vi "Main.vi"() -> ()   [LabVIEW 2018] (continued)
            n2414 = Not(x=w322) -> (.not. x?=→"ST90通讯状态":bool)
            n2415 = Index Array(array=w319, index=0 ("索引")) -> (element=w320:u32)
            n2416 = Number To Boolean Array(number=w320) -> (Boolean array=w321:bool[])
            n2417 = Index Array(array=w321, index #1=0 ("索引")) -> (element #1=w285:bool, element #2=w284:bool, element #3=w283:bool, element #4=w282:bool, element #5=w278:bool)  [unwired: 4 in]
            "ST901扫码请求" <- w285
            "ST901数据读取" <- w284
            "ST902扫码请求" <- w282
            "ST902数据读取" <- w278
            "ST901编码请求" <- w283
            n2418 = call <vilib>:"Boolean Crossing PtByPt.vi"("direction"=enum16{"either", "false-true", "true-false"}."false-true", "input"=w285) -> ("crossing"=w307:bool)  [unwired: 1 in]
            n2419 = disable-structure shown="启用" {
              disable-tunnel: [w334 w336] -> w294
              disable-tunnel: w285 -> [w333 w336]
              frame Disabled {
                n2420 = call <vilib>:"Boolean Crossing PtByPt.vi"("direction"=enum16{"either", "false-true", "true-false"}."true-false", "input"=w333) -> ("crossing"=w334:bool)  [unwired: 1 in]
              }
              frame Enabled {
              }
            }
            n2421 = case shown="真" w307 {
              tunnel: w309 -> [w513 w518]
              tunnel: w308 -> [w512 w519]
              tunnel: [w513 w517] -> w306
              tunnel: [w512 w515] -> w305
              frame False {
              }
              frame True {
                w527 = u16 0 items=["byte", "word", "Dword"] ("数据类型")
                w525 = u8 132 items=["I/O (P)"=128, "Input (I)"=129, "Output (Q)"=130, "Bit Memory (M)"=131, "Data (DB)"=132, "Instance Data (DI)"=133, "Local Data (L)"=134, "Predecessor Local Data (VL)"=135] ("寄存器类型")
                n2422 = call "S7_Read.vi"("TCP"=w518, "DB #"=u16 20, "读取长度"=u16 13, "寄存器类型"=w525, "起始地址"=u32 6, "数据类型"=w527, "error in"=w519) -> ("TCP"=w517:refnum<k5>, "数据"=w522:u32[], "error out"=w520:errorcluster)  [unwired: 5 in, 1 out]
                n2423 = To Unsigned Word Integer(number=w522) -> (unsigned 16bit integer=w521:u16[])
                n2424 = call "还原为字符串.vi"("error in (no error)"=w520, "输入数组"=w521) -> ("error out"=w516:errorcluster, "字符串"=w514:string)  [unwired: 8 in]
                n2425 = stacked-sequence {
                  tunnel: w516 -> [_ w531]
                  tunnel: [_ w530] -> w515
                  tunnel: w514 -> [w528 _]
                  frame #0 {
                    "901二维码" <- w528
                  }
                  frame #1 {
                    n2426 = property on="ST901扫码请求（事件）" class="Bool (严格)"(error in=w531, "Val(Sgnl)"=TRUE ("值(信号)")) -> (error out=w530:errorcluster)  [unwired: 1 in, 1 out]
                  }
                }
              }
            }
            n2427 = case shown="假" w294 {
              frame False {
                n2428 = local write "901扫码回复输入"(FALSE ("301扫码回复输入")) -> ()
              }
              frame True {
              }
            }
            n2429 = call <vilib>:"Boolean Crossing PtByPt.vi"("direction"=enum16{"either", "false-true", "true-false"}."false-true", "input"=w284) -> ("crossing"=w303:bool)  [unwired: 1 in]
            n2430 = disable-structure shown="启用" {
              disable-tunnel: enum16{"either", "false-true", "true-false"}."true-false" ("direction") -> [w343 _]
              disable-tunnel: [w342 w344] -> w300
              disable-tunnel: w284 -> [w341 w344]
              frame Disabled {
                n2431 = call <vilib>:"Boolean Crossing PtByPt.vi"("direction"=w343, "input"=w341) -> ("crossing"=w342:bool)  [unwired: 1 in]
              }
              frame Enabled {
              }
            }
            n2432 = case shown="真" w303 {
              tunnel: [w443 w460] -> w298
              tunnel: [w442 w445] -> w297
              tunnel: w305 -> [w442 w470]
              tunnel: w306 -> [w443 w471]
              frame False {
              }
              frame True {
                w467 = u16 2 items=["byte", "word", "Dword"] ("数据类型")
                w465 = u8 132 items=["I/O (P)"=128, "Input (I)"=129, "Output (Q)"=130, "Bit Memory (M)"=131, "Data (DB)"=132, "Instance Data (DI)"=133, "Local Data (L)"=134, "Predecessor Local Data (VL)"=135] ("寄存器类型")
                w480 = u16 2 items=["byte", "word", "Dword"] ("数据类型")
                w482 = u8 132 items=["I/O (P)"=128, "Input (I)"=129, "Output (Q)"=130, "Bit Memory (M)"=131, "Data (DB)"=132, "Instance Data (DI)"=133, "Local Data (L)"=134, "Predecessor Local Data (VL)"=135] ("寄存器类型")
                w475 = u16 1 items=["byte", "word", "Dword"] ("数据类型")
                w477 = u8 132 items=["I/O (P)"=128, "Input (I)"=129, "Output (Q)"=130, "Bit Memory (M)"=131, "Data (DB)"=132, "Instance Data (DI)"=133, "Local Data (L)"=134, "Predecessor Local Data (VL)"=135] ("寄存器类型")
                n2433 = call "S7_Read.vi"("TCP"=w471, "DB #"=u16 20, "读取长度"=u16 1, "寄存器类型"=w477, "起始地址"=u32 82, "数据类型"=w475, "error in"=w470) -> ("TCP"=w488:refnum<k5>, "数据"=w490:u32[], "error out"=w489:errorcluster)  [unwired: 5 in, 1 out]
                n2434 = Index Array(array=w490) -> (element=w492:u32)  [unwired: 1 in]
                n2435 = Equal?(x=w492, y=u32 1) -> (x = y?=w491:bool)
                n2436 = case shown="真" w491 {
                  tunnel: ["NG" "OK"] -> w469
                  frame False {
                  }
                  frame True {
                  }
                }
                n2437 = call "S7_Read.vi"("TCP"=w488, "DB #"=u16 20, "读取长度"=u16 12, "寄存器类型"=w482, "起始地址"=u32 34, "数据类型"=w480, "error in"=w489) -> ("TCP"=w462:refnum<k5>, "数据"=w458:u32[], "error out"=w461:errorcluster)  [unwired: 5 in, 1 out]
                n2438 = Divide(x=w458, y=u32[] [100, 100, 100, 100, 100, 100, 100, 100, 100, 100, 100, 100]) -> (x/y=w457:dbl[])
                n2439 = Number To Fractional String(number=w457, precision (6)=i16 2 ("精度(6)")) -> (F-format string=w468:string[])  [unwired: 2 in]
                n2440 = call "S7_Read.vi"("TCP"=w462, "DB #"=u16 20, "读取长度"=u16 9, "寄存器类型"=w465, "起始地址"=u32 100, "数据类型"=w467, "error in"=w461) -> ("TCP"=w460:refnum<k5>, "数据"=w454:u32[], "error out"=w459:errorcluster)  [unwired: 5 in, 1 out]
                n2441 = Divide(x=w454, y=u32[] [100, 100, 1000, 1000, 1000, 1000, 1000, 1000, 1000]) -> (x/y=w452:dbl[])
                n2442 = Delete From Array(array=w452, length=2 ("长度"), index=0 ("索引")) -> (deleted portion=w448:dbl[], array with subset deleted=w449:dbl[])
                n2443 = for {
                  tunnel: w449 -> [w509] mode=indexing
                  tunnel: [w508] -> w446 mode=indexing
                  n2444 = Number To Fractional String(number=w509, precision (6)=i16 3 ("精度(6)")) -> (F-format string=w508:string)  [unwired: 2 in]
                }
                n2445 = for {
                  tunnel: w448 -> [w506] mode=indexing
                  tunnel: [w504] -> w447 mode=indexing
                  n2446 = Number To Fractional String(number=w506, precision (6)=i16 2 ("精度(6)")) -> (F-format string=w504:string)  [unwired: 2 in]
                }
                n2447 = Format Date/Time String(time format string (%c)="%Y-%m-%d" ("时间格式字符串(%c)")) -> (date/time string=w493:string)  [unwired: 2 in]
                n2448 = Get Date/Time String(want seconds? (F)=TRUE ("需要秒？(F)")) -> (time string=w494:string)  [unwired: 2 in, 1 out]
                n2449 = Insert Into Array(array=string[] [] ("数组"), index=0 ("索引"), new element #1="901" ("新元素/子数组"), new element #2=w469, new element #3=w493, new element #4=w494, new element #5=w469, new element #6=w468, new element #7=w447, new element #8=w446) -> (w444:string[])
                n2450 = stacked-sequence {
                  tunnel: w459 -> [_ w499]
                  tunnel: [_ w496] -> w445
                  tunnel: w444 -> [w495 _]
                  frame #0 {
                    "901数据" <- w495
                  }
                  frame #1 {
                    n2451 = property on="ST901数据读取（事件）" class="Bool (严格)"(error in=w499, "Val(Sgnl)"=TRUE ("值(信号)")) -> (error out=w497:errorcluster)  [unwired: 1 in, 1 out]
                    n2452 = disable-structure shown="禁用" {
                      disable-tunnel: w497 -> [w501 w503]
                      disable-tunnel: [w500 w503] -> w496
                      frame Disabled {
                        n2453 = property on="ST90画曲线" class="Bool (严格)"(error in=w501, "Val(Sgnl)"=TRUE ("值(信号)")) -> (error out=w500:errorcluster)  [unwired: 1 in, 1 out]
                      }
                      frame Enabled {
                      }
                    }
                  }
                }
              }
            }
            n2454 = case shown="假" w300 {
              frame False {
                n2455 = local write "901数据回复输入"(FALSE ("301数据回复输入")) -> ()
              }
              frame True {
              }
            }
            n2456 = disable-structure shown="启用" {
              disable-tunnel: [w331 w332] -> w299
              disable-tunnel: w283 -> [w329 w332]
              frame Disabled {
                n2457 = call <vilib>:"Boolean Crossing PtByPt.vi"("direction"=enum16{"either", "false-true", "true-false"}."true-false", "input"=w329) -> ("crossing"=w331:bool)  [unwired: 1 in]
              }
              frame Enabled {
              }
            }
            n2458 = case shown="假" w299 {
              frame False {
                n2459 = local write "901编码回复输入"(FALSE ("302扫码回复输入")) -> ()
              }
              frame True {
              }
            }
            n2460 = disable-structure shown="启用" {
              disable-tunnel: [w326 w328] -> w287
              disable-tunnel: w282 -> [w325 w328]
              frame Disabled {
                n2461 = call <vilib>:"Boolean Crossing PtByPt.vi"("direction"=enum16{"either", "false-true", "true-false"}."true-false", "input"=w325) -> ("crossing"=w326:bool)  [unwired: 1 in]
              }
              frame Enabled {
              }
            }
            n2462 = case shown="假" w287 {
              frame False {
                n2463 = local write "902扫码回复输入"(FALSE ("302数据回复输入")) -> ()
              }
              frame True {
              }
            }
            n2464 = disable-structure shown="启用" {
              disable-tunnel: [w339 w340] -> w286
              disable-tunnel: w278 -> [w337 w340]
              frame Disabled {
                n2465 = call <vilib>:"Boolean Crossing PtByPt.vi"("direction"=enum16{"either", "false-true", "true-false"}."true-false", "input"=w337) -> ("crossing"=w339:bool)  [unwired: 1 in]
              }
              frame Enabled {
              }
            }
            n2466 = case shown="假" w286 {
              frame False {
                n2467 = local write "902数据回复输入"(FALSE ("303扫码回复输入")) -> ()
              }
              frame True {
              }
            }
            n2468 = call <vilib>:"Boolean Crossing PtByPt.vi"("direction"=enum16{"either", "false-true", "true-false"}."false-true", "input"=w283) -> ("crossing"=w296:bool)  [unwired: 1 in]
            n2469 = case shown="真" w296 {
              tunnel: w298 -> [w411 w420]
              tunnel: w297 -> [w410 w419]
              tunnel: [w410 w416] -> w281
              tunnel: [w411 w418] -> w280
              frame False {
              }
              frame True {
                w421 = u16 0 items=["byte", "word", "Dword"] ("数据类型")
                w423 = u8 132 items=["I/O (P)"=128, "Input (I)"=129, "Output (Q)"=130, "Bit Memory (M)"=131, "Data (DB)"=132, "Instance Data (DI)"=133, "Local Data (L)"=134, "Predecessor Local Data (VL)"=135] ("寄存器类型")
                n2470 = call "S7_Read.vi"("TCP"=w420, "DB #"=u16 20, "读取长度"=u16 14, "寄存器类型"=w423, "起始地址"=u32 84, "数据类型"=w421, "error in"=w419) -> ("TCP"=w418:refnum<k5>, "数据"=w426:u32[], "error out"=w428:errorcluster)  [unwired: 5 in, 1 out]
                n2471 = To Unsigned Word Integer(number=w426) -> (unsigned 16bit integer=w427:u16[])
                n2472 = call "还原为字符串.vi"("error in (no error)"=w428, "输入数组"=w427) -> ("error out"=w417:errorcluster, "字符串"=w413:string)  [unwired: 8 in]
                n2473 = String To Byte Array(string=w413) -> (unsigned byte array=w414:u8[])
                n2474 = for {
                  tunnel: w414 -> [w434] mode=indexing
                  tunnel: [w433] -> w415 mode=indexing
                  n2475 = Equal?(x=w434, y=u8 32) -> (x = y?=w435:bool)
                  n2476 = case shown="真" w435 {
                    tunnel: w434 -> [w437 _]
                    tunnel: [w437 u8 48] -> w433
                    frame False {
                    }
                    frame True {
                    }
                  }
                }
                n2477 = Byte Array To String(unsigned byte array=w415) -> (string=w412:string)
                n2478 = stacked-sequence {
                  tunnel: w417 -> [_ w432]
                  tunnel: [_ w431] -> w416
                  tunnel: w412 -> [w429 _]
                  frame #0 {
                    "901编码" <- w429
                  }
                  frame #1 {
                    n2479 = property on="ST901编码请求 （事件）" class="Bool (严格)"(error in=w432, "Val(Sgnl)"=TRUE ("值(信号)")) -> (error out=w431:errorcluster)  [unwired: 1 in, 1 out]
                  }
                }
              }
            }
            n2480 = call <vilib>:"Boolean Crossing PtByPt.vi"("direction"=enum16{"either", "false-true", "true-false"}."false-true", "input"=w282) -> ("crossing"=w279:bool)  [unwired: 1 in]
            n2481 = case shown="真" w279 {
              tunnel: w280 -> [w391 w397]
              tunnel: w281 -> [w390 w396]
              tunnel: [w390 w393] -> w290
              tunnel: [w391 w395] -> w277
              frame False {
              }
              frame True {
                w398 = u16 0 items=["byte", "word", "Dword"] ("数据类型")
                w400 = u8 132 items=["I/O (P)"=128, "Input (I)"=129, "Output (Q)"=130, "Bit Memory (M)"=131, "Data (DB)"=132, "Instance Data (DI)"=133, "Local Data (L)"=134, "Predecessor Local Data (VL)"=135] ("寄存器类型")
                n2482 = call "S7_Read.vi"("TCP"=w397, "DB #"=u16 20, "读取长度"=u16 13, "寄存器类型"=w400, "起始地址"=u32 146, "数据类型"=w398, "error in"=w396) -> ("TCP"=w395:refnum<k5>, "数据"=w403:u32[], "error out"=w405:errorcluster)  [unwired: 5 in, 1 out]
                n2483 = To Unsigned Word Integer(number=w403) -> (unsigned 16bit integer=w404:u16[])
                n2484 = call "还原为字符串.vi"("error in (no error)"=w405, "输入数组"=w404) -> ("error out"=w394:errorcluster, "字符串"=w392:string)  [unwired: 8 in]
                n2485 = stacked-sequence {
                  tunnel: w394 -> [_ w409]
                  tunnel: [_ w408] -> w393
                  tunnel: w392 -> [w406 _]
                  frame #0 {
                    "902二维码" <- w406
                  }
                  frame #1 {
                    n2486 = property on="ST902扫码请求（事件）" class="Bool (严格)"(error in=w409, "Val(Sgnl)"=TRUE ("值(信号)")) -> (error out=w408:errorcluster)  [unwired: 1 in, 1 out]
                  }
                }
              }
            }
            n2487 = call <vilib>:"Boolean Crossing PtByPt.vi"("direction"=enum16{"either", "false-true", "true-false"}."false-true", "input"=w278) -> ("crossing"=w291:bool)  [unwired: 1 in]
            n2488 = case shown="真" w291 {
              tunnel: w277 -> [w348 w358]
              tunnel: w290 -> [w347 w357]
              tunnel: [w348 w359] -> w289
              tunnel: [w347 w355] -> w288
              frame False {
              }
              frame True {
                w365 = u16 1 items=["byte", "word", "Dword"] ("数据类型")
                w367 = u8 132 items=["I/O (P)"=128, "Input (I)"=129, "Output (Q)"=130, "Bit Memory (M)"=131, "Data (DB)"=132, "Instance Data (DI)"=133, "Local Data (L)"=134, "Predecessor Local Data (VL)"=135] ("寄存器类型")
                w360 = u16 2 items=["byte", "word", "Dword"] ("数据类型")
                w362 = u8 132 items=["I/O (P)"=128, "Input (I)"=129, "Output (Q)"=130, "Bit Memory (M)"=131, "Data (DB)"=132, "Instance Data (DI)"=133, "Local Data (L)"=134, "Predecessor Local Data (VL)"=135] ("寄存器类型")
                n2489 = call "S7_Read.vi"("TCP"=w358, "DB #"=u16 20, "读取长度"=u16 3, "寄存器类型"=w362, "起始地址"=u32 160, "数据类型"=w360, "error in"=w357) -> ("TCP"=w376:refnum<k5>, "数据"=w354:u32[], "error out"=w377:errorcluster)  [unwired: 5 in, 1 out]
                n2490 = Divide(x=w354, y=u32[] [1000, 1000, 1000]) -> (x/y=w352:dbl[])
                n2491 = Number To Fractional String(number=w352, precision (6)=i16 3 ("精度(6)")) -> (F-format string=w350:string[])  [unwired: 2 in]
                n2492 = call "S7_Read.vi"("TCP"=w376, "DB #"=u16 20, "读取长度"=u16 1, "寄存器类型"=w367, "起始地址"=u32 172, "数据类型"=w365, "error in"=w377) -> ("TCP"=w359:refnum<k5>, "数据"=w378:u32[], "error out"=w356:errorcluster)  [unwired: 5 in, 1 out]
                n2493 = Index Array(array=w378) -> (element=w380:u32)  [unwired: 1 in]
                n2494 = Equal?(x=w380, y=u32 1) -> (x = y?=w379:bool)
                n2495 = case shown="真" w379 {
                  tunnel: ["NG" "OK"] -> w383
                  frame False {
                  }
                  frame True {
                  }
                }
                n2496 = Format Date/Time String(time format string (%c)="%Y-%m-%d" ("时间格式字符串(%c)")) -> (date/time string=w381:string)  [unwired: 2 in]
                n2497 = Get Date/Time String(want seconds? (F)=TRUE ("需要秒？(F)")) -> (time string=w382:string)  [unwired: 2 in, 1 out]
                n2498 = Insert Into Array(array=string[] [] ("数组"), index=0 ("索引"), new element #1="902" ("新元素/子数组"), new element #2=w383, new element #3=w381, new element #4=w382, new element #5=w383, new element #6=w350) -> (w349:string[])
                n2499 = stacked-sequence {
                  tunnel: w356 -> [_ w387]
                  tunnel: [_ w386] -> w355
                  tunnel: w349 -> [w384 _]
                  frame #0 {
                    "902数据" <- w384
                  }
                  frame #1 {
                    n2500 = property on="ST902数据读取（事件）" class="Bool (严格)"(error in=w387, "Val(Sgnl)"=TRUE ("值(信号)")) -> (error out=w386:errorcluster)  [unwired: 1 in, 1 out]
                  }
                }
              }
            }
          }
          frame "写" {
            w551 = u8 132 items=["I/O (P)"=128, "Input (I)"=129, "Output (Q)"=130, "Bit Memory (M)"=131, "Data (DB)"=132, "Instance Data (DI)"=133, "Local Data (L)"=134, "Predecessor Local Data (VL)"=135] ("寄存器类型")
            w550 = u16 1 items=["byte", "word", "Dword"] ("数据类型")
            w544 = u8 132 items=["I/O (P)"=128, "Input (I)"=129, "Output (Q)"=130, "Bit Memory (M)"=131, "Data (DB)"=132, "Instance Data (DI)"=133, "Local Data (L)"=134, "Predecessor Local Data (VL)"=135] ("寄存器类型")
            w543 = u16 1 items=["byte", "word", "Dword"] ("数据类型")
            w565 = u8 132 items=["I/O (P)"=128, "Input (I)"=129, "Output (Q)"=130, "Bit Memory (M)"=131, "Data (DB)"=132, "Instance Data (DI)"=133, "Local Data (L)"=134, "Predecessor Local Data (VL)"=135] ("寄存器类型")
            w564 = u16 1 items=["byte", "word", "Dword"] ("数据类型")
            w578 = u8 132 items=["I/O (P)"=128, "Input (I)"=129, "Output (Q)"=130, "Bit Memory (M)"=131, "Data (DB)"=132, "Instance Data (DI)"=133, "Local Data (L)"=134, "Predecessor Local Data (VL)"=135] ("寄存器类型")
            w579 = u16 1 items=["byte", "word", "Dword"] ("数据类型")
            w581 = u8 132 items=["I/O (P)"=128, "Input (I)"=129, "Output (Q)"=130, "Bit Memory (M)"=131, "Data (DB)"=132, "Instance Data (DI)"=133, "Local Data (L)"=134, "Predecessor Local Data (VL)"=135] ("寄存器类型")
            w580 = u16 1 items=["byte", "word", "Dword"] ("数据类型")
            w588 = u8 132 items=["I/O (P)"=128, "Input (I)"=129, "Output (Q)"=130, "Bit Memory (M)"=131, "Data (DB)"=132, "Instance Data (DI)"=133, "Local Data (L)"=134, "Predecessor Local Data (VL)"=135] ("寄存器类型")
            w585 = u16 1 items=["byte", "word", "Dword"] ("数据类型")
            n2501 = local read "90看门狗"() -> (w558:i32)
            n2502 = case shown="0" w558 {
              tunnel: [0 ("y") 1 ("y")] -> w557
              frame 1, Default {
              }
              frame 0 {
              }
            }
            "90看门狗" <- w557
            n2503 = call "S7_Write.vi"("TCP"=w584, "寄存器类型"=w588, "DB #"=u16 20, "写入地址"=u32 32, "数据类型"=w585, "写入数据"=w557) -> ("TCP"=w572:refnum<k5>, "error out"=w571:errorcluster)  [unwired: 7 in, 1 out]
            n2504 = case shown="真" "901扫码回复输入" {
              tunnel: w572 -> [w637 w645]
              tunnel: w571 -> [w636 w644]
              tunnel: [w637 w643] -> w570
              tunnel: [w636 w642] -> w569
              tunnel: [999 w641] -> w568
              frame False {
              }
              frame True {
                w653 = u8 132 items=["I/O (P)"=128, "Input (I)"=129, "Output (Q)"=130, "Bit Memory (M)"=131, "Data (DB)"=132, "Instance Data (DI)"=133, "Local Data (L)"=134, "Predecessor Local Data (VL)"=135] ("寄存器类型")
                w652 = u16 1 items=["byte", "word", "Dword"] ("数据类型")
                w647 = u8 132 items=["I/O (P)"=128, "Input (I)"=129, "Output (Q)"=130, "Bit Memory (M)"=131, "Data (DB)"=132, "Instance Data (DI)"=133, "Local Data (L)"=134, "Predecessor Local Data (VL)"=135] ("寄存器类型")
                w648 = u16 1 items=["byte", "word", "Dword"] ("数据类型")
                n2505 = local read "上一站号 (901)"() -> (w640:string)
                n2506 = local read "上一站结果 (901)"() -> (w639:string)
                n2507 = Decimal String To Number(string=w640, default (0L)=u32 0 ("默认(0 I32)")) -> (number=w657:u32)  [unwired: 1 in, 1 out]
                n2508 = call "S7_Write.vi"("TCP"=w645, "寄存器类型"=w647, "DB #"=u16 20, "写入地址"=u32 28, "数据类型"=w648, "写入数据"=w657, "error in"=w644) -> ("TCP"=w656:refnum<k5>, "error out"=w655:errorcluster)  [unwired: 6 in, 1 out]
                n2509 = Equal?(x=w639, y="OK") -> (x = y?=w659:bool)
                n2510 = case shown="假" w659 {
                  tunnel: [u32 2 ("写入数据") u32 1 ("写入数据")] -> w660
                  frame False {
                  }
                  frame True {
                  }
                }
                n2511 = local read "扫码请求回复901"() -> (w638:string)
                n2512 = call "S7_Write.vi"("TCP"=w656, "寄存器类型"=w653, "DB #"=u16 20, "写入地址"=u32 30, "数据类型"=w652, "写入数据"=w660, "error in"=w655) -> ("TCP"=w643:refnum<k5>, "error out"=w642:errorcluster)  [unwired: 6 in, 1 out]
                n2513 = Decimal String To Number(string=w638) -> (number=w641:i32)  [unwired: 2 in, 1 out]
              }
            }
            n2514 = call "S7_Write.vi"("TCP"=w570, "寄存器类型"=w581, "DB #"=u16 20, "写入地址"=u32 2, "数据类型"=w580, "写入数据"=w568, "error in"=w569) -> ("TCP"=w563:refnum<k5>, "error out"=w562:errorcluster)  [unwired: 6 in, 1 out]
            n2515 = case shown="真" "901数据回复输入" {
              tunnel: [999 w634] -> w561
              frame False {
              }
              frame True {
                n2516 = local read "数据保存请求回复901"() -> (w633:string)
                n2517 = Decimal String To Number(string=w633) -> (number=w634:i32)  [unwired: 2 in, 1 out]
              }
            }
            n2518 = call "S7_Write.vi"("TCP"=w563, "寄存器类型"=w565, "DB #"=u16 20, "写入地址"=u32 4, "数据类型"=w564, "写入数据"=w561, "error in"=w562) -> ("TCP"=w560:refnum<k5>, "error out"=w559:errorcluster)  [unwired: 6 in, 1 out]
            n2519 = case shown="真" "901编码回复输入" {
              tunnel: [999 w669] -> w575
              tunnel: w560 -> [w664 w683]
              tunnel: w559 -> [w663 w682]
              tunnel: [w664 w671] -> w574
              tunnel: [w663 w670] -> w573
              frame False {
              }
              frame True {
                w677 = u8 132 items=["I/O (P)"=128, "Input (I)"=129, "Output (Q)"=130, "Bit Memory (M)"=131, "Data (DB)"=132, "Instance Data (DI)"=133, "Local Data (L)"=134, "Predecessor Local Data (VL)"=135] ("寄存器类型")
                w678 = u16 1 items=["byte", "word", "Dword"] ("数据类型")
                w685 = u8 132 items=["I/O (P)"=128, "Input (I)"=129, "Output (Q)"=130, "Bit Memory (M)"=131, "Data (DB)"=132, "Instance Data (DI)"=133, "Local Data (L)"=134, "Predecessor Local Data (VL)"=135] ("寄存器类型")
                w684 = u16 1 items=["byte", "word", "Dword"] ("数据类型")
                n2520 = local read "上一站号 (901) 编码"() -> (w668:string)
                n2521 = Decimal String To Number(string=w668) -> (number=w681:i32)  [unwired: 2 in, 1 out]
                n2522 = local read "上一站结果 (901)编码"() -> (w667:string)
                n2523 = call "S7_Write.vi"("TCP"=w683, "寄存器类型"=w685, "DB #"=u16 20, "写入地址"=u32 22, "数据类型"=w684, "写入数据"=w681, "error in"=w682) -> ("TCP"=w673:refnum<k5>, "error out"=w674:errorcluster)  [unwired: 6 in, 1 out]
                n2524 = local read "编码请求回复901"() -> (w666:string)
                n2525 = Equal?(x=w667, y="OK") -> (x = y?=w680:bool)
                n2526 = case shown="假" w680 {
                  tunnel: [u32 2 ("写入数据") u32 1 ("写入数据")] -> w672
                  frame False {
                  }
                  frame True {
                  }
                }
                n2527 = call "S7_Write.vi"("TCP"=w673, "寄存器类型"=w677, "DB #"=u16 20, "写入地址"=u32 24, "数据类型"=w678, "写入数据"=w672, "error in"=w674) -> ("TCP"=w671:refnum<k5>, "error out"=w670:errorcluster)  [unwired: 6 in, 1 out]
                n2528 = Decimal String To Number(string=w666) -> (number=w669:i32)  [unwired: 2 in, 1 out]
              }
            }
            n2529 = call "S7_Write.vi"("TCP"=w574, "寄存器类型"=w578, "DB #"=u16 20, "写入地址"=u32 20, "数据类型"=w579, "写入数据"=w575, "error in"=w573) -> ("TCP"=w540:refnum<k5>, "error out"=w539:errorcluster)  [unwired: 6 in, 1 out]
            n2530 = case shown="假" "902扫码回复输入" {
              tunnel: [999 w611] -> w547
              tunnel: w540 -> [w606 w625]
              tunnel: w539 -> [w605 w624]
              tunnel: [w606 w613] -> w548
              tunnel: [w605 w612] -> w549
              frame False {
              }
              frame True {
                w619 = u8 132 items=["I/O (P)"=128, "Input (I)"=129, "Output (Q)"=130, "Bit Memory (M)"=131, "Data (DB)"=132, "Instance Data (DI)"=133, "Local Data (L)"=134, "Predecessor Local Data (VL)"=135] ("寄存器类型")
                w620 = u16 1 items=["byte", "word", "Dword"] ("数据类型")
                w627 = u8 132 items=["I/O (P)"=128, "Input (I)"=129, "Output (Q)"=130, "Bit Memory (M)"=131, "Data (DB)"=132, "Instance Data (DI)"=133, "Local Data (L)"=134, "Predecessor Local Data (VL)"=135] ("寄存器类型")
                w626 = u16 1 items=["byte", "word", "Dword"] ("数据类型")
                n2531 = local read "上一站号 (902)"() -> (w610:string)
                n2532 = Decimal String To Number(string=w610) -> (number=w623:i32)  [unwired: 2 in, 1 out]
                n2533 = call "S7_Write.vi"("TCP"=w625, "寄存器类型"=w627, "DB #"=u16 20, "写入地址"=u32 142, "数据类型"=w626, "写入数据"=w623, "error in"=w624) -> ("TCP"=w615:refnum<k5>, "error out"=w616:errorcluster)  [unwired: 6 in, 1 out]
                n2534 = local read "上一站结果 (902)"() -> (w609:string)
                n2535 = local read "扫码请求回复902"() -> (w608:string)
                n2536 = Equal?(x=w609, y="OK") -> (x = y?=w622:bool)
                n2537 = case shown="假" w622 {
                  tunnel: [u32 2 ("写入数据") u32 1 ("写入数据")] -> w614
                  frame False {
                  }
                  frame True {
                  }
                }
                n2538 = call "S7_Write.vi"("TCP"=w615, "寄存器类型"=w619, "DB #"=u16 20, "写入地址"=u32 144, "数据类型"=w620, "写入数据"=w614, "error in"=w616) -> ("TCP"=w613:refnum<k5>, "error out"=w612:errorcluster)  [unwired: 6 in, 1 out]
                n2539 = Decimal String To Number(string=w608) -> (number=w611:i32)  [unwired: 2 in, 1 out]
              }
            }
            n2540 = call "S7_Write.vi"("TCP"=w548, "寄存器类型"=w544, "DB #"=u16 20, "写入地址"=u32 138, "数据类型"=w543, "写入数据"=w547, "error in"=w549) -> ("TCP"=w555:refnum<k5>, "error out"=w554:errorcluster)  [unwired: 6 in, 1 out]
            n2541 = case shown="真" "902数据回复输入" {
              tunnel: [999 w604] -> w556
              frame False {
              }
              frame True {
                n2542 = local read "数据保存请求回复902"() -> (w603:string)
                n2543 = Decimal String To Number(string=w603) -> (number=w604:i32)  [unwired: 2 in, 1 out]
              }
            }
            n2544 = call "S7_Write.vi"("TCP"=w555, "寄存器类型"=w551, "DB #"=u16 20, "写入地址"=u32 140, "数据类型"=w550, "写入数据"=w556, "error in"=w554) -> ("TCP"=w535:refnum<k5>, "error out"=w534:errorcluster)  [unwired: 6 in, 1 out]
            n2545 = disable-structure shown="启用" {
              disable-tunnel: w535 -> [w591 w595]
              disable-tunnel: [w591 w598] -> w533
              disable-tunnel: w534 -> [w592 w596]
              disable-tunnel: [w592 w597] -> w532
              frame Disabled {
              }
              frame Enabled {
                w600 = u8 132 items=["I/O (P)"=128, "Input (I)"=129, "Output (Q)"=130, "Bit Memory (M)"=131, "Data (DB)"=132, "Instance Data (DI)"=133, "Local Data (L)"=134, "Predecessor Local Data (VL)"=135] ("寄存器类型")
                w594 = u16 1 items=["byte", "word", "Dword"] ("数据类型")
                n2546 = local read "产品型号"() -> (w593:u32)
                n2547 = call "S7_Write.vi"("TCP"=w595, "寄存器类型"=w600, "DB #"=u16 20, "写入地址"=u32 174, "数据类型"=w594, "写入数据"=w593, "error in"=w596) -> ("TCP"=w598:refnum<k5>, "error out"=w597:errorcluster)  [unwired: 6 in, 1 out]
              }
            }
          }
          frame "错误" {
            n2548 = call "S7_Close.vi"("TCP Connection Ref"=w694) -> ("error out"=w695:errorcluster)  [unwired: 10 in]
            n2549 = call <vilib>:"Clear Errors.vi"("error in (no error)"=w695) -> ()  [unwired: 5 in, 2 out]
          }
          frame "退出" {
            n2550 = call "S7_Close.vi"("TCP Connection Ref"=w701) -> ("error out"=w702:errorcluster)  [unwired: 10 in]
            n2551 = call <vilib>:"Clear Errors.vi"("error in (no error)"=w702) -> ()  [unwired: 5 in, 2 out]
          }
        }
      }
      n2552 = while {
        shift-right: [w2983] -> _
        shift-left: errorcluster {"status"=FALSE, "code"=0, "source"=""} ("错误常量") -> [w2986]
        shift-right: [w2982] -> _
        shift-left: enum16{"初始化", "读", "写", "错误", "退出"}."初始化" -> [w2987]
        shift-right: [w2984] -> _
        shift-left: _ -> [w2981]
        stop <- w2980 stop-if-true
        n2553 = local read "退出"() -> (w2988:bool)
        n2554 = case shown="假" w2988 {
          tunnel: w2987 -> [w2989 _]
          tunnel: [w2990 enum16{"初始化", "读", "写", "错误", "退出"}."退出"] -> w2979
          tunnel: w2986 -> [w2991 _]
          frame False {
            n2555 = case shown="错误" w2991 {
              tunnel: [w2992 enum16{"初始化", "读", "写", "错误", "退出"}."错误"] -> w2990
              tunnel: w2989 -> [w2992 _]
              frame No Error {
              }
              frame Error {
              }
            }
          }
          frame True {
          }
        }
        n2556 = Wait (ms)(milliseconds to wait=u32 80 ("等待时间（毫秒）")) -> ()  [unwired: 1 out]
        n2557 = case shown="\"写\"" w2979 {
          tunnel: [w2997 w3048 w3357 refnum<k5> refnum ("TCP") refnum<k5> refnum ("TCP")] -> w2984
          tunnel: [w2995 w3047 w3356 errorcluster {"status"=FALSE, "code"=0, "source"=""} ("error out") errorcluster {"status"=FALSE, "code"=0, "source"=""} ("error out")] -> w2983
          tunnel: [enum16{"初始化", "读", "写", "错误", "退出"}."读" enum16{"初始化", "读", "写", "错误", "退出"}."写" enum16{"初始化", "读", "写", "错误", "退出"}."读" enum16{"初始化", "读", "写", "错误", "退出"}."初始化" enum16{"初始化", "读", "写", "错误", "退出"}."退出"] -> w2982
          tunnel: w2981 -> [_ w3080 w3416 w3529 w3536]
          tunnel: [FALSE FALSE FALSE FALSE TRUE] -> w2980
          frame "初始化", Default {
            w3022 = u16 0 items=["byte", "word", "Dword"] ("数据类型")
            w3024 = u8 132 items=["I/O (P)"=128, "Input (I)"=129, "Output (Q)"=130, "Bit Memory (M)"=131, "Data (DB)"=132, "Instance Data (DI)"=133, "Local Data (L)"=134, "Predecessor Local Data (VL)"=135] ("寄存器类型")
            w3014 = u16 0 items=["byte", "word", "Dword"] ("数据类型")
            w3016 = u8 132 items=["I/O (P)"=128, "Input (I)"=129, "Output (Q)"=130, "Bit Memory (M)"=131, "Data (DB)"=132, "Instance Data (DI)"=133, "Local Data (L)"=134, "Predecessor Local Data (VL)"=135] ("寄存器类型")
            w3013 = u16 0 items=["byte", "word", "Dword"] ("数据类型")
            w3011 = u8 132 items=["I/O (P)"=128, "Input (I)"=129, "Output (Q)"=130, "Bit Memory (M)"=131, "Data (DB)"=132, "Instance Data (DI)"=133, "Local Data (L)"=134, "Predecessor Local Data (VL)"=135] ("寄存器类型")
            w3034 = u8 0 items=["S7-1200.200.200SMART"=0, "S7-300"=2, "S7-400"=3] ("PLC 系列")
            n2558 = call "S7_Open.vi"("IP 地址"="192.168.1.30", "PLC 系列"=w3034, "超时（MS）"=100) -> ("TCP"=w2998:refnum<k5>, "error out"=w2996:errorcluster)  [unwired: 10 in, 1 out]
            n2559 = case shown="错误" w2996 {
              tunnel: [FALSE TRUE] -> w3030
              frame No Error {
              }
              frame Error {
              }
            }
            n2560 = local write "ST30通讯状态"(w3030) -> ()
            n2561 = call "S7_Read.vi"("TCP"=w2998, "DB #"=u16 20, "读取长度"=u16 13, "寄存器类型"=w3011, "起始地址"=u32 30, "数据类型"=w3013, "error in"=w2996) -> ("TCP"=w3004:refnum<k5>, "数据"=w3008:u32[], "error out"=w3006:errorcluster)  [unwired: 5 in, 1 out]
            n2562 = To Unsigned Word Integer(number=w3008) -> (unsigned 16bit integer=w3007:u16[])
            n2563 = call "还原为字符串.vi"("error in (no error)"=w3006, "输入数组"=w3007) -> ("error out"=w3003:errorcluster, "字符串"=w3005:string)  [unwired: 8 in]
            n2564 = local write "301二维码"(w3005) -> ()
            n2565 = call "S7_Read.vi"("TCP"=w3004, "DB #"=u16 20, "读取长度"=u16 13, "寄存器类型"=w3016, "起始地址"=u32 52, "数据类型"=w3014, "error in"=w3003) -> ("TCP"=w3001:refnum<k5>, "数据"=w3019:u32[], "error out"=w3021:errorcluster)  [unwired: 5 in, 1 out]
            n2566 = To Unsigned Word Integer(number=w3019) -> (unsigned 16bit integer=w3020:u16[])
            n2567 = call "还原为字符串.vi"("error in (no error)"=w3021, "输入数组"=w3020) -> ("error out"=w3000:errorcluster, "字符串"=w3002:string)  [unwired: 8 in]
            n2568 = local write "302二维码"(w3002) -> ()
            n2569 = call "S7_Read.vi"("TCP"=w3001, "DB #"=u16 20, "读取长度"=u16 13, "寄存器类型"=w3024, "起始地址"=u32 74, "数据类型"=w3022, "error in"=w3000) -> ("TCP"=w2997:refnum<k5>, "数据"=w3027:u32[], "error out"=w3029:errorcluster)  [unwired: 5 in, 1 out]
            n2570 = To Unsigned Word Integer(number=w3027) -> (unsigned 16bit integer=w3028:u16[])
            n2571 = call "还原为字符串.vi"("error in (no error)"=w3029, "输入数组"=w3028) -> ("error out"=w2995:errorcluster, "字符串"=w2999:string)  [unwired: 8 in]
            n2572 = local write "303二维码"(w2999) -> ()
          }
          frame "读" {
            w3081 = u16 0 items=["byte", "word", "Dword"] ("数据类型")
            w3083 = u8 132 items=["I/O (P)"=128, "Input (I)"=129, "Output (Q)"=130, "Bit Memory (M)"=131, "Data (DB)"=132, "Instance Data (DI)"=133, "Local Data (L)"=134, "Predecessor Local Data (VL)"=135] ("寄存器类型")
            # "6"
            # "11"
            n2573 = call "S7_Read.vi"("TCP"=w3080, "DB #"=u16 20, "读取长度"=u16 1, "寄存器类型"=w3083, "起始地址"=u32 0, "数据类型"=w3081) -> ("TCP"=w3078:refnum<k5>, "数据"=w3088:u32[], "读取成功"=w3091:bool, "error out"=w3077:errorcluster)  [unwired: 6 in]
            n2574 = Not(x=w3091) -> (.not. x?=→"ST30通讯状态":bool)
            n2575 = Index Array(array=w3088, index=0 ("索引")) -> (element=w3089:u32)
            n2576 = Number To Boolean Array(number=w3089) -> (Boolean array=w3090:bool[])
            n2577 = Index Array(array=w3090, index #1=0 ("索引"), index #7=7 ("索引")) -> (element #1=w3059:bool, element #2=w3046:bool, element #3=w3045:bool, element #4=w3042:bool, element #5=w3041:bool, element #6=w3038:bool, element #7=w3049:bool)  [unwired: 5 in]
            "ST301扫码请求" <- w3059
            "ST301数据读取" <- w3046
            "ST302扫码请求" <- w3045
            "ST302数据读取" <- w3042
            "ST303扫码请求" <- w3041
            "ST303数据读取" <- w3038
            n2578 = disable-structure shown="启用" {
              disable-tunnel: [w3103 w3105] -> w3061
              disable-tunnel: w3059 -> [w3102 w3105]
              frame Disabled {
                n2579 = call <vilib>:"Boolean Crossing PtByPt.vi"("direction"=enum16{"either", "false-true", "true-false"}."true-false", "input"=w3102) -> ("crossing"=w3103:bool)  [unwired: 1 in]
              }
              frame Enabled {
              }
            }
            n2580 = call <vilib>:"Boolean Crossing PtByPt.vi"("direction"=enum16{"either", "false-true", "true-false"}."false-true", "input"=w3059) -> ("crossing"=w3076:bool)  [unwired: 1 in]
            n2581 = case shown="真" w3076 {
              tunnel: w3078 -> [w3337 w3342]
              tunnel: w3077 -> [w3336 w3343]
              tunnel: [w3337 w3341] -> w3075
              tunnel: [w3336 w3339] -> w3074
              frame False {
              }
              frame True {
                w3351 = u16 0 items=["byte", "word", "Dword"] ("数据类型")
                w3349 = u8 132 items=["I/O (P)"=128, "Input (I)"=129, "Output (Q)"=130, "Bit Memory (M)"=131, "Data (DB)"=132, "Instance Data (DI)"=133, "Local Data (L)"=134, "Predecessor Local Data (VL)"=135] ("寄存器类型")
                n2582 = call "S7_Read.vi"("TCP"=w3342, "DB #"=u16 20, "读取长度"=u16 13, "寄存器类型"=w3349, "起始地址"=u32 30, "数据类型"=w3351, "error in"=w3343) -> ("TCP"=w3341:refnum<k5>, "数据"=w3346:u32[], "error out"=w3344:errorcluster)  [unwired: 5 in, 1 out]
                n2583 = To Unsigned Word Integer(number=w3346) -> (unsigned 16bit integer=w3345:u16[])
                n2584 = call "还原为字符串.vi"("error in (no error)"=w3344, "输入数组"=w3345) -> ("error out"=w3340:errorcluster, "字符串"=w3338:string)  [unwired: 8 in]
                n2585 = stacked-sequence {
                  tunnel: w3340 -> [_ w3355]
                  tunnel: [_ w3354] -> w3339
                  tunnel: w3338 -> [w3352 _]
                  frame #0 {
                    "301二维码" <- w3352
                  }
                  frame #1 {
                    n2586 = property on="ST301扫码请求 (事件)" class="Bool (严格)"(error in=w3355, "Val(Sgnl)"=TRUE ("值(信号)")) -> (error out=w3354:errorcluster)  [unwired: 1 in, 1 out]
                  }
                }
              }
            }
            n2587 = case shown="假" w3061 {
              frame False {
                n2588 = local write "301扫码回复输入"(FALSE ("301扫码回复输入")) -> ()
              }
              frame True {
              }
            }
            n2589 = disable-structure shown="启用" {
              disable-tunnel: [w3115 w3117] -> w3070
              disable-tunnel: w3046 -> [w3114 w3117]
              frame Disabled {
                n2590 = call <vilib>:"Boolean Crossing PtByPt.vi"("direction"=enum16{"either", "false-true", "true-false"}."true-false", "input"=w3114) -> ("crossing"=w3115:bool)  [unwired: 1 in]
              }
              frame Enabled {
              }
            }
            n2591 = call <vilib>:"Boolean Crossing PtByPt.vi"("direction"=enum16{"either", "false-true", "true-false"}."false-true", "input"=w3046) -> ("crossing"=w3072:bool)  [unwired: 1 in]
            n2592 = case shown="真" w3072 {
              tunnel: [w3280 w3295] -> w3068
              tunnel: [w3279 w3286] -> w3067
              tunnel: w3074 -> [w3279 w3296]
              tunnel: w3075 -> [w3280 w3297]
              tunnel: w3049 -> [_ w3289]
              frame False {
              }
              frame True {
                w3311 = u16 1 items=["byte", "word", "Dword"] ("数据类型")
                w3313 = u8 132 items=["I/O (P)"=128, "Input (I)"=129, "Output (Q)"=130, "Bit Memory (M)"=131, "Data (DB)"=132, "Instance Data (DI)"=133, "Local Data (L)"=134, "Predecessor Local Data (VL)"=135] ("寄存器类型")
                w3306 = u16 1 items=["byte", "word", "Dword"] ("数据类型")
                w3308 = u8 132 items=["I/O (P)"=128, "Input (I)"=129, "Output (Q)"=130, "Bit Memory (M)"=131, "Data (DB)"=132, "Instance Data (DI)"=133, "Local Data (L)"=134, "Predecessor Local Data (VL)"=135] ("寄存器类型")
                w3301 = u16 1 items=["byte", "word", "Dword"] ("数据类型")
                w3303 = u8 132 items=["I/O (P)"=128, "Input (I)"=129, "Output (Q)"=130, "Bit Memory (M)"=131, "Data (DB)"=132, "Instance Data (DI)"=133, "Local Data (L)"=134, "Predecessor Local Data (VL)"=135] ("寄存器类型")
                n2593 = case shown="真" w3289 {
                  tunnel: ["F" "T"] -> w3288
                  frame False {
                  }
                  frame True {
                  }
                }
                n2594 = call "S7_Read.vi"("TCP"=w3297, "DB #"=u16 20, "读取长度"=u16 4, "寄存器类型"=w3303, "起始地址"=u32 96, "数据类型"=w3301, "error in"=w3296) -> ("TCP"=w3319:refnum<k5>, "数据"=w3285:u32[], "error out"=w3320:errorcluster)  [unwired: 5 in, 1 out]
                n2595 = Divide(x=w3285, y=u32[] [100, 100, 100, 100]) -> (x/y=w3283:dbl[])
                n2596 = Number To Fractional String(number=w3283, precision (6)=i16 2 ("精度(6)")) -> (F-format string=w3291:string[])  [unwired: 2 in]
                n2597 = call "S7_Read.vi"("TCP"=w3319, "DB #"=u16 20, "读取长度"=u16 1, "寄存器类型"=w3308, "起始地址"=u32 94, "数据类型"=w3306, "error in"=w3320) -> ("TCP"=w3321:refnum<k5>, "数据"=w3323:u32[], "error out"=w3322:errorcluster)  [unwired: 5 in, 1 out]
                n2598 = Index Array(array=w3323) -> (element=w3325:u32)  [unwired: 1 in]
                n2599 = Equal?(x=w3325, y=u32 1) -> (x = y?=w3324:bool)
                n2600 = case shown="真" w3324 {
                  tunnel: ["NG" "OK"] -> w3290
                  frame False {
                  }
                  frame True {
                  }
                }
                n2601 = call "S7_Read.vi"("TCP"=w3321, "DB #"=u16 20, "读取长度"=u16 1, "寄存器类型"=w3313, "起始地址"=u32 104, "数据类型"=w3311, "error in"=w3322) -> ("TCP"=w3295:refnum<k5>, "数据"=w3294:u32[], "error out"=w3287:errorcluster)  [unwired: 5 in, 1 out]
                n2602 = Index Array(array=w3294) -> (element=w3293:u32)  [unwired: 1 in]
                n2603 = Number To Decimal String(number=w3293) -> (decimal integer string=w3292:string)  [unwired: 1 in]
                n2604 = Format Date/Time String(time format string (%c)="%Y-%m-%d" ("时间格式字符串(%c)")) -> (date/time string=w3326:string)  [unwired: 2 in]
                n2605 = Get Date/Time String(want seconds? (F)=TRUE ("需要秒？(F)")) -> (time string=w3327:string)  [unwired: 2 in, 1 out]
                n2606 = Insert Into Array(array=string[] [] ("数组"), index=0 ("索引"), new element #1="301" ("新元素/子数组"), new element #2=w3290, new element #3=w3326, new element #4=w3327, new element #5=w3288, new element #6=w3290, new element #7=w3291, new element #8=w3292) -> (w3281:string[])
                n2607 = stacked-sequence {
                  tunnel: w3287 -> [_ w3331]
                  tunnel: [_ w3330] -> w3286
                  tunnel: w3281 -> [w3328 _]
                  frame #0 {
                    "301数据" <- w3328
                  }
                  frame #1 {
                    n2608 = property on="ST301数据读取 (事件)" class="Bool (严格)"(error in=w3331, "Val(Sgnl)"=TRUE ("值(信号)")) -> (error out=w3330:errorcluster)  [unwired: 1 in, 1 out]
                  }
                }
              }
            }
            n2609 = case shown="假" w3070 {
              frame False {
                n2610 = local write "301数据回复输入"(FALSE ("301数据回复输入")) -> ()
              }
              frame True {
              }
            }
            n2611 = disable-structure shown="启用" {
              disable-tunnel: [w3100 w3101] -> w3069
              disable-tunnel: w3045 -> [w3098 w3101]
              frame Disabled {
                n2612 = call <vilib>:"Boolean Crossing PtByPt.vi"("direction"=enum16{"either", "false-true", "true-false"}."true-false", "input"=w3098) -> ("crossing"=w3100:bool)  [unwired: 1 in]
              }
              frame Enabled {
              }
            }
            n2613 = case shown="假" w3069 {
              frame False {
                n2614 = local write "302扫码回复输入"(FALSE ("302扫码回复输入")) -> ()
              }
              frame True {
              }
            }
            n2615 = disable-structure shown="启用" {
              disable-tunnel: [w3111 w3113] -> w3044
              disable-tunnel: w3042 -> [w3110 w3113]
              frame Disabled {
                n2616 = call <vilib>:"Boolean Crossing PtByPt.vi"("direction"=enum16{"either", "false-true", "true-false"}."true-false", "input"=w3110) -> ("crossing"=w3111:bool)  [unwired: 1 in]
              }
              frame Enabled {
              }
            }
            n2617 = case shown="假" w3044 {
              frame False {
                n2618 = local write "302数据回复输入"(FALSE ("302数据回复输入")) -> ()
              }
              frame True {
              }
            }
            n2619 = disable-structure shown="启用" {
              disable-tunnel: [w3096 w3097] -> w3043
              disable-tunnel: w3041 -> [w3094 w3097]
              frame Disabled {
                n2620 = call <vilib>:"Boolean Crossing PtByPt.vi"("direction"=enum16{"either", "false-true", "true-false"}."true-false", "input"=w3094) -> ("crossing"=w3096:bool)  [unwired: 1 in]
              }
              frame Enabled {
              }
            }
            n2621 = case shown="假" w3043 {
              frame False {
                n2622 = local write "303扫码回复输入"(FALSE ("303扫码回复输入")) -> ()
              }
              frame True {
              }
            }
            n2623 = call <vilib>:"Boolean Crossing PtByPt.vi"("direction"=enum16{"either", "false-true", "true-false"}."false-true", "input"=w3045) -> ("crossing"=w3066:bool)  [unwired: 1 in]
            n2624 = case shown="真" w3066 {
              tunnel: w3068 -> [w3257 w3263]
              tunnel: w3067 -> [w3256 w3262]
              tunnel: [w3256 w3259] -> w3064
              tunnel: [w3257 w3261] -> w3065
              frame False {
              }
              frame True {
                w3264 = u16 0 items=["byte", "word", "Dword"] ("数据类型")
                w3266 = u8 132 items=["I/O (P)"=128, "Input (I)"=129, "Output (Q)"=130, "Bit Memory (M)"=131, "Data (DB)"=132, "Instance Data (DI)"=133, "Local Data (L)"=134, "Predecessor Local Data (VL)"=135] ("寄存器类型")
                n2625 = call "S7_Read.vi"("TCP"=w3263, "DB #"=u16 20, "读取长度"=u16 13, "寄存器类型"=w3266, "起始地址"=u32 52, "数据类型"=w3264, "error in"=w3262) -> ("TCP"=w3261:refnum<k5>, "数据"=w3269:u32[], "error out"=w3271:errorcluster)  [unwired: 5 in, 1 out]
                n2626 = To Unsigned Word Integer(number=w3269) -> (unsigned 16bit integer=w3270:u16[])
                n2627 = call "还原为字符串.vi"("error in (no error)"=w3271, "输入数组"=w3270) -> ("error out"=w3260:errorcluster, "字符串"=w3258:string)  [unwired: 8 in]
                n2628 = stacked-sequence {
                  tunnel: w3260 -> [_ w3275]
                  tunnel: [_ w3274] -> w3259
                  tunnel: w3258 -> [w3272 _]
                  frame #0 {
                    "302二维码" <- w3272
                  }
                  frame #1 {
                    n2629 = property on="ST302扫码请求 (事件)" class="Bool (严格)"(error in=w3275, "Val(Sgnl)"=TRUE ("值(信号)")) -> (error out=w3274:errorcluster)  [unwired: 1 in, 1 out]
                  }
                }
              }
            }
            n2630 = disable-structure shown="启用" {
              disable-tunnel: enum16{"either", "false-true", "true-false"}."true-false" ("direction") -> [w3108 _]
              disable-tunnel: [w3107 w3109] -> w3039
              disable-tunnel: w3038 -> [w3106 w3109]
              frame Disabled {
                n2631 = call <vilib>:"Boolean Crossing PtByPt.vi"("direction"=w3108, "input"=w3106) -> ("crossing"=w3107:bool)  [unwired: 1 in]
              }
              frame Enabled {
              }
            }
            n2632 = case shown="假" w3039 {
              frame False {
                n2633 = local write "303数据回复输入"(FALSE ("303数据回复输入")) -> ()
              }
              frame True {
              }
            }
            n2634 = call <vilib>:"Boolean Crossing PtByPt.vi"("direction"=enum16{"either", "false-true", "true-false"}."false-true", "input"=w3042) -> ("crossing"=w3062:bool)  [unwired: 1 in]
            n2635 = case shown="真" w3062 {
              tunnel: w3065 -> [w3216 w3222]
              tunnel: w3064 -> [w3215 w3221]
              tunnel: [w3216 w3220] -> w3055
              tunnel: [w3215 w3218] -> w3054
              frame False {
              }
              frame True {
                w3228 = u16 1 items=["byte", "word", "Dword"] ("数据类型")
                w3230 = u8 132 items=["I/O (P)"=128, "Input (I)"=129, "Output (Q)"=130, "Bit Memory (M)"=131, "Data (DB)"=132, "Instance Data (DI)"=133, "Local Data (L)"=134, "Predecessor Local Data (VL)"=135] ("寄存器类型")
                w3223 = u16 1 items=["byte", "word", "Dword"] ("数据类型")
                w3225 = u8 132 items=["I/O (P)"=128, "Input (I)"=129, "Output (Q)"=130, "Bit Memory (M)"=131, "Data (DB)"=132, "Instance Data (DI)"=133, "Local Data (L)"=134, "Predecessor Local Data (VL)"=135] ("寄存器类型")
                n2636 = call "S7_Read.vi"("TCP"=w3222, "DB #"=u16 20, "读取长度"=u16 1, "寄存器类型"=w3225, "起始地址"=u32 106, "数据类型"=w3223, "error in"=w3221) -> ("TCP"=w3239:refnum<k5>, "数据"=w3241:u32[], "error out"=w3240:errorcluster)  [unwired: 5 in, 1 out]
                n2637 = Index Array(array=w3241) -> (element=w3242:u32)  [unwired: 1 in]
                n2638 = Number To Decimal String(number=w3242) -> (decimal integer string=w3249:string)  [unwired: 1 in]
                n2639 = call "S7_Read.vi"("TCP"=w3239, "DB #"=u16 20, "读取长度"=u16 1, "寄存器类型"=w3230, "起始地址"=u32 110, "数据类型"=w3228, "error in"=w3240) -> ("TCP"=w3220:refnum<k5>, "数据"=w3243:u32[], "error out"=w3219:errorcluster)  [unwired: 5 in, 1 out]
                n2640 = Index Array(array=w3243) -> (element=w3245:u32)  [unwired: 1 in]
                n2641 = Equal?(x=w3245, y=u32 1) -> (x = y?=w3244:bool)
                n2642 = case shown="真" w3244 {
                  tunnel: ["NG" "OK"] -> w3248
                  frame False {
                  }
                  frame True {
                  }
                }
                n2643 = Format Date/Time String(time format string (%c)="%Y-%m-%d" ("时间格式字符串(%c)")) -> (date/time string=w3246:string)  [unwired: 2 in]
                n2644 = Get Date/Time String(want seconds? (F)=TRUE ("需要秒？(F)")) -> (time string=w3247:string)  [unwired: 2 in, 1 out]
                n2645 = Insert Into Array(array=string[] [] ("数组"), index=0 ("索引"), new element #1="302" ("新元素/子数组"), new element #2=w3248, new element #3=w3246, new element #4=w3247, new element #5=w3248, new element #6=w3249) -> (w3217:string[])
                n2646 = stacked-sequence {
                  tunnel: w3219 -> [_ w3253]
                  tunnel: [_ w3252] -> w3218
                  tunnel: w3217 -> [w3250 _]
                  frame #0 {
                    "302data" <- w3250
                  }
                  frame #1 {
                    n2647 = property on="ST302数据读取 (事件)" class="Bool (严格)"(error in=w3253, "Val(Sgnl)"=TRUE ("值(信号)")) -> (error out=w3252:errorcluster)  [unwired: 1 in, 1 out]
                  }
                }
              }
            }
            n2648 = call <vilib>:"Boolean Crossing PtByPt.vi"("direction"=enum16{"either", "false-true", "true-false"}."false-true", "input"=w3041) -> ("crossing"=w3057:bool)  [unwired: 1 in]
            n2649 = case shown="真" w3057 {
              tunnel: w3055 -> [w3196 w3202]
              tunnel: w3054 -> [w3195 w3201]
              tunnel: [w3195 w3198] -> w3050
              tunnel: [w3196 w3200] -> w3051
              frame False {
              }
              frame True {
                w3203 = u16 0 items=["byte", "word", "Dword"] ("数据类型")
                w3205 = u8 132 items=["I/O (P)"=128, "Input (I)"=129, "Output (Q)"=130, "Bit Memory (M)"=131, "Data (DB)"=132, "Instance Data (DI)"=133, "Local Data (L)"=134, "Predecessor Local Data (VL)"=135] ("寄存器类型")
                n2650 = call "S7_Read.vi"("TCP"=w3202, "DB #"=u16 20, "读取长度"=u16 13, "寄存器类型"=w3205, "起始地址"=u32 74, "数据类型"=w3203, "error in"=w3201) -> ("TCP"=w3200:refnum<k5>, "数据"=w3208:u32[], "error out"=w3210:errorcluster)  [unwired: 5 in, 1 out]
                n2651 = To Unsigned Word Integer(number=w3208) -> (unsigned 16bit integer=w3209:u16[])
                n2652 = call "还原为字符串.vi"("error in (no error)"=w3210, "输入数组"=w3209) -> ("error out"=w3199:errorcluster, "字符串"=w3197:string)  [unwired: 8 in]
                n2653 = stacked-sequence {
                  tunnel: w3199 -> [_ w3214]
                  tunnel: [_ w3213] -> w3198
                  tunnel: w3197 -> [w3211 _]
                  frame #0 {
                    "303二维码" <- w3211
                  }
                  frame #1 {
                    n2654 = property on="ST303扫码请求 (事件)" class="Bool (严格)"(error in=w3214, "Val(Sgnl)"=TRUE ("值(信号)")) -> (error out=w3213:errorcluster)  [unwired: 1 in, 1 out]
                  }
                }
              }
            }
            n2655 = call <vilib>:"Boolean Crossing PtByPt.vi"("direction"=enum16{"either", "false-true", "true-false"}."false-true", "input"=w3038) -> ("crossing"=w3052:bool)  [unwired: 1 in]
            n2656 = case shown="真" w3052 {
              tunnel: w3051 -> [w3122 w3152]
              tunnel: w3050 -> [w3121 w3153]
              tunnel: [w3122 w3161] -> w3048
              tunnel: [w3121 w3159] -> w3047
              frame False {
              }
              frame True {
                w3148 = 15 ("长度")
                w3158 = u16 0 items=["byte", "word", "Dword"] ("数据类型")
                w3156 = u8 132 items=["I/O (P)"=128, "Input (I)"=129, "Output (Q)"=130, "Bit Memory (M)"=131, "Data (DB)"=132, "Instance Data (DI)"=133, "Local Data (L)"=134, "Predecessor Local Data (VL)"=135] ("寄存器类型")
                w3167 = u16 1 items=["byte", "word", "Dword"] ("数据类型")
                w3169 = u8 132 items=["I/O (P)"=128, "Input (I)"=129, "Output (Q)"=130, "Bit Memory (M)"=131, "Data (DB)"=132, "Instance Data (DI)"=133, "Local Data (L)"=134, "Predecessor Local Data (VL)"=135] ("寄存器类型")
                w3162 = u16 1 items=["byte", "word", "Dword"] ("数据类型")
                w3164 = u8 132 items=["I/O (P)"=128, "Input (I)"=129, "Output (Q)"=130, "Bit Memory (M)"=131, "Data (DB)"=132, "Instance Data (DI)"=133, "Local Data (L)"=134, "Predecessor Local Data (VL)"=135] ("寄存器类型")
                n2657 = call "S7_Read.vi"("TCP"=w3152, "DB #"=u16 20, "读取长度"=u16 60, "寄存器类型"=w3156, "起始地址"=u32 114, "数据类型"=w3158, "error in"=w3153) -> ("TCP"=w3128:refnum<k5>, "数据"=w3147:u32[], "error out"=w3127:errorcluster)  [unwired: 5 in, 1 out]
                n2658 = Delete From Array(array=w3147, length=w3148, index=2 ("索引")) -> (deleted portion=w3131:u32[])  [unwired: 1 out]
                n2659 = Delete From Array(array=w3147, length=w3148, index=22 ("索引")) -> (deleted portion=w3130:u32[])  [unwired: 1 out]
                n2660 = Delete From Array(array=w3147, length=w3148, index=42 ("索引")) -> (deleted portion=w3129:u32[])  [unwired: 1 out]
                n2661 = To Unsigned Word Integer(number=w3130) -> (unsigned 16bit integer=w3141:u16[])
                n2662 = To Unsigned Word Integer(number=w3131) -> (unsigned 16bit integer=w3132:u16[])
                n2663 = To Unsigned Word Integer(number=w3129) -> (unsigned 16bit integer=w3146:u16[])
                n2664 = call "还原为字符串.vi"("输入数组"=w3132) -> ("字符串"=w3134:string)  [unwired: 9 in, 1 out]
                n2665 = call "还原为字符串.vi"("输入数组"=w3141) -> ("字符串"=w3139:string)  [unwired: 9 in, 1 out]
                n2666 = call "还原为字符串.vi"("输入数组"=w3146) -> ("字符串"=w3144:string)  [unwired: 9 in, 1 out]
                n2667 = Match Pattern(string=w3134, regular expression="\r" ("正则表达式")) -> (before substring=w3133:string)  [unwired: 1 in, 3 out]
                n2668 = Match Pattern(string=w3139, regular expression="\r" ("正则表达式")) -> (before substring=w3140:string)  [unwired: 1 in, 3 out]
                n2669 = Match Pattern(string=w3144, regular expression="\r" ("正则表达式")) -> (before substring=w3145:string)  [unwired: 1 in, 3 out]
                n2670 = Match Pattern(string=w3133, regular expression="\u0000" ("正则表达式")) -> (before substring=w3126:string)  [unwired: 1 in, 3 out]
                n2671 = Match Pattern(string=w3140, regular expression="\u0000" ("正则表达式")) -> (before substring=w3125:string)  [unwired: 1 in, 3 out]
                n2672 = Match Pattern(string=w3145, regular expression="\u0000" ("正则表达式")) -> (before substring=w3124:string)  [unwired: 1 in, 3 out]
                n2673 = call "S7_Read.vi"("TCP"=w3128, "DB #"=u16 20, "读取长度"=u16 1, "寄存器类型"=w3164, "起始地址"=u32 108, "数据类型"=w3162, "error in"=w3127) -> ("TCP"=w3178:refnum<k5>, "数据"=w3180:u32[], "error out"=w3179:errorcluster)  [unwired: 5 in, 1 out]
                n2674 = Index Array(array=w3180) -> (element=w3181:u32)  [unwired: 1 in]
                n2675 = Number To Decimal String(number=w3181) -> (decimal integer string=w3188:string)  [unwired: 1 in]
                n2676 = call "S7_Read.vi"("TCP"=w3178, "DB #"=u16 20, "读取长度"=u16 1, "寄存器类型"=w3169, "起始地址"=u32 112, "数据类型"=w3167, "error in"=w3179) -> ("TCP"=w3161:refnum<k5>, "数据"=w3182:u32[], "error out"=w3160:errorcluster)  [unwired: 5 in, 1 out]
                n2677 = Index Array(array=w3182) -> (element=w3184:u32)  [unwired: 1 in]
                n2678 = Equal?(x=w3184, y=u32 1) -> (x = y?=w3183:bool)
                n2679 = case shown="真" w3183 {
                  tunnel: ["NG" "OK"] -> w3187
                  frame False {
                  }
                  frame True {
                  }
                }
                n2680 = Format Date/Time String(time format string (%c)="%Y-%m-%d" ("时间格式字符串(%c)")) -> (date/time string=w3185:string)  [unwired: 2 in]
                n2681 = Get Date/Time String(want seconds? (F)=TRUE ("需要秒？(F)")) -> (time string=w3186:string)  [unwired: 2 in, 1 out]
                n2682 = Insert Into Array(array=string[] [] ("数组"), index=0 ("索引"), new element #1="303" ("新元素/子数组"), new element #2=w3187, new element #3=w3185, new element #4=w3186, new element #5=w3187, new element #6=w3188, new element #7=w3126, new element #8=w3125, new element #9=w3124) -> (w3123:string[])
                n2683 = stacked-sequence {
                  tunnel: w3160 -> [_ w3192]
                  tunnel: [_ w3191] -> w3159
                  tunnel: w3123 -> [w3189 _]
                  frame #0 {
                    "303data" <- w3189
                  }
                  frame #1 {
                    n2684 = property on="ST303数据读取 (事件)" class="Bool (严格)"(error in=w3192, "Val(Sgnl)"=TRUE ("值(信号)")) -> (error out=w3191:errorcluster)  [unwired: 1 in, 1 out]
                  }
                }
              }
            }
          }
          frame "写" {
            w3372 = u8 132 items=["I/O (P)"=128, "Input (I)"=129, "Output (Q)"=130, "Bit Memory (M)"=131, "Data (DB)"=132, "Instance Data (DI)"=133, "Local Data (L)"=134, "Predecessor Local Data (VL)"=135] ("寄存器类型")
            w3371 = u16 1 items=["byte", "word", "Dword"] ("数据类型")
            w3365 = u8 132 items=["I/O (P)"=128, "Input (I)"=129, "Output (Q)"=130, "Bit Memory (M)"=131, "Data (DB)"=132, "Instance Data (DI)"=133, "Local Data (L)"=134, "Predecessor Local Data (VL)"=135] ("寄存器类型")
            w3364 = u16 1 items=["byte", "word", "Dword"] ("数据类型")
            w3390 = u8 132 items=["I/O (P)"=128, "Input (I)"=129, "Output (Q)"=130, "Bit Memory (M)"=131, "Data (DB)"=132, "Instance Data (DI)"=133, "Local Data (L)"=134, "Predecessor Local Data (VL)"=135] ("寄存器类型")
            w3389 = u16 1 items=["byte", "word", "Dword"] ("数据类型")
            w3403 = u8 132 items=["I/O (P)"=128, "Input (I)"=129, "Output (Q)"=130, "Bit Memory (M)"=131, "Data (DB)"=132, "Instance Data (DI)"=133, "Local Data (L)"=134, "Predecessor Local Data (VL)"=135] ("寄存器类型")
            w3404 = u16 1 items=["byte", "word", "Dword"] ("数据类型")
            w3410 = u8 132 items=["I/O (P)"=128, "Input (I)"=129, "Output (Q)"=130, "Bit Memory (M)"=131, "Data (DB)"=132, "Instance Data (DI)"=133, "Local Data (L)"=134, "Predecessor Local Data (VL)"=135] ("寄存器类型")
            w3411 = u16 1 items=["byte", "word", "Dword"] ("数据类型")
            w3413 = u8 132 items=["I/O (P)"=128, "Input (I)"=129, "Output (Q)"=130, "Bit Memory (M)"=131, "Data (DB)"=132, "Instance Data (DI)"=133, "Local Data (L)"=134, "Predecessor Local Data (VL)"=135] ("寄存器类型")
            w3412 = u16 1 items=["byte", "word", "Dword"] ("数据类型")
            w3420 = u8 132 items=["I/O (P)"=128, "Input (I)"=129, "Output (Q)"=130, "Bit Memory (M)"=131, "Data (DB)"=132, "Instance Data (DI)"=133, "Local Data (L)"=134, "Predecessor Local Data (VL)"=135] ("寄存器类型")
            w3417 = u16 1 items=["byte", "word", "Dword"] ("数据类型")
            n2685 = local read "30看门狗"() -> (w3383:i32)
            n2686 = case shown="0" w3383 {
              tunnel: [0 ("y") 1 ("y")] -> w3382
              frame 1, Default {
              }
              frame 0 {
              }
            }
            "30看门狗" <- w3382
            n2687 = call "S7_Write.vi"("TCP"=w3416, "寄存器类型"=w3420, "DB #"=u16 20, "写入地址"=u32 2, "数据类型"=w3417, "写入数据"=w3382) -> ("TCP"=w3397:refnum<k5>, "error out"=w3396:errorcluster)  [unwired: 7 in, 1 out]
            n2688 = case shown="真" "301扫码回复输入" {
              tunnel: w3397 -> [w3469 w3477]
              tunnel: w3396 -> [w3468 w3476]
              tunnel: [w3469 w3475] -> w3395
              tunnel: [w3468 w3474] -> w3394
              tunnel: [999 w3473] -> w3393
              frame False {
              }
              frame True {
                w3485 = u8 132 items=["I/O (P)"=128, "Input (I)"=129, "Output (Q)"=130, "Bit Memory (M)"=131, "Data (DB)"=132, "Instance Data (DI)"=133, "Local Data (L)"=134, "Predecessor Local Data (VL)"=135] ("寄存器类型")
                w3484 = u16 1 items=["byte", "word", "Dword"] ("数据类型")
